vi "Save Error.vi"(4 "Error In (no error)":errorcluster, 7 "Source":string) -> (0 "error out":errorcluster)   [LabVIEW 2023]
doc: "Ver 1:00\nDESCRIPTION\nFormats and saves error\n\nERROR HANDLING\nPass out file error\n---------------------------------\nVERSION CONTROL\nVer 1:00 07/04/2000 ssdc"
uses:
  ErrordBCommand.ctl
panel:
  # "Local"
  # "Input"
  # "Output"
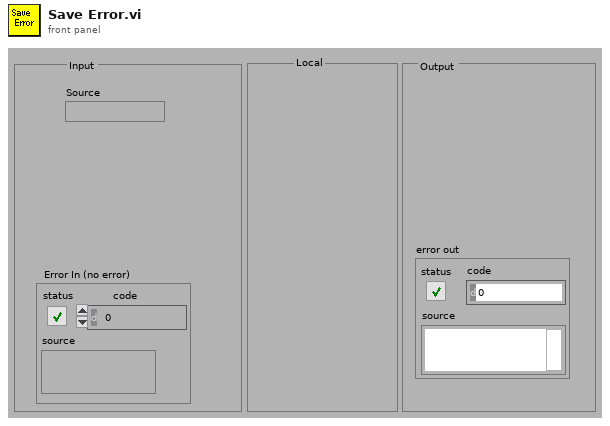
[diagram p1: front panel]
types:
  T1 = typedef "ErrordBCommand.ctl" = enum16{"No Command - Error", "Get All Errors", "Get #Errors", "Clear Error Log", "Insert New Error", "Update Existing Error"}
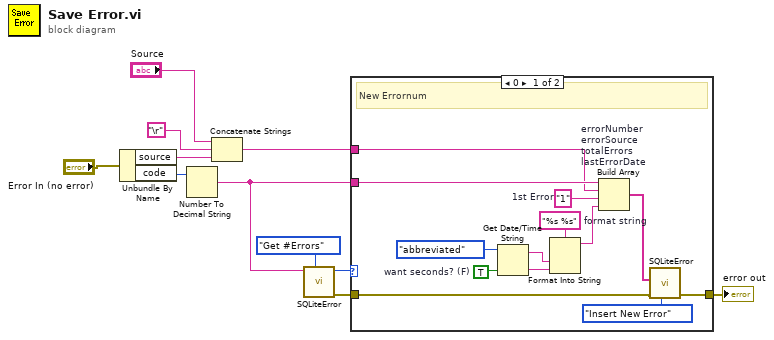
[diagram p0: block diagram]
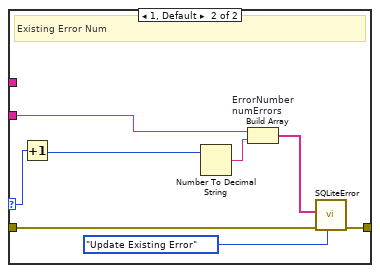
[diagram p2: hidden frame]
diagram:
  n1 = Unbundle By Name("Error In (no error)") -> ("source"=w6:string, "code"=w10:i32)
  n2 = Number To Decimal String(number=w10) -> (decimal integer string=w7:string)  [unwired: 1 in]
  n3 = Concatenate Strings("Source", "\r", w6) -> (w4:string)
  n4 = call "SQLiteError.vi"("ConfigCommand"=ErrordBCommand."Get #Errors", "ErrorNumber"=w7) -> ("error out"=w8:errorcluster, "#Errors"=w9:i32)  [unwired: 4 in, 1 out]
  n5 = case shown="0" w9 {
    selector: w9 -> [_ w27]
    tunnel: w7 -> [w21 w32]
    tunnel: w8 -> [w22 w31]
    tunnel: [w23 w29] -> w2
    tunnel: w4 -> [w19 _]
    frame 0 {
      w16 = "%s %s"  # format string
      w12 = TRUE  # want seconds? (F)
      w18 = "1"  # 1st Error
      # "New Errornum"
      n6 = Get Date/Time String(date format (0)=enum16{"short", "long", "abbreviated"}."abbreviated", want seconds? (F)=w12) -> (date string=w15:string, time string=w14:string)  [unwired: 1 in]
      n7 = Format Into String(format string=w16, w15, w14) -> (resulting string=w13:string)  [unwired: 2 in, 1 out]
      n8 = Build Array "errorNumber\nerrorSource\ntotalErrors\nlastErrorDate"(w21, w19, w18, w13) -> (w20:string[])
      n9 = call "SQLiteError.vi"("ConfigCommand"=ErrordBCommand."Insert New Error", "error in (no error)"=w22, "ErrorData"=w20) -> ("error out"=w23:errorcluster)  [unwired: 3 in, 2 out]
    }
    frame 1, Default {
      # "Existing Error Num"
      n10 = Increment(x=w27) -> (x+1=w26:i32)
      n11 = Number To Decimal String(number=w26) -> (decimal integer string=w25:string)  [unwired: 1 in]
      n12 = Build Array "ErrorNumber\nnumErrors"(w32, w25) -> (w28:string[])
      n13 = call "SQLiteError.vi"("ConfigCommand"=ErrordBCommand."Update Existing Error", "error in (no error)"=w31, "ErrorData"=w28) -> ("error out"=w29:errorcluster)  [unwired: 3 in, 2 out]
    }
  }
  "error out" <- w2
